vi "Serial_Init.vi"(8 "error in (no error)":errorcluster, 10 "input cluster":T1={"baud rate (9600)"=115200, "data bits (8)"=8, "parity (0:none)"=enum."None", "stop bits (10: 1 bit)"=10, "flow control (0:none)"=0, "termination char\n(0xA = '\\n' = LF) "=10, "Enable Termination\nChar (T)"=TRUE, "timeout (10sec)"=10000} {"termination char\n(0xA = '\\n' = LF)" format="%.0x"; "flow control (0:none)" items=["None", "XON/XOFF", "RTS/CTS", "XON/XOFF & RTS/CTS", "DTR/DSR", "XON/XOFF & DTR/DSR"]; "stop bits (10: 1 bit)" items=["1.0"=10, "1.5"=15, "2.0"=20]; "data bits (8)" min=5 max=8 step=1}, 11 "VISA Refnum in":refnum<visa-resource-name>="ASRL1::INSTR") -> (0 "error out":errorcluster, 1 "timeout (10sec)":u32=10000, 2 "Bytes at Port":u32, 3 "VISA Refnum out":refnum<visa-resource-name>)   [LabVIEW 2017]
uses:
  <vilib>/myRIO/Instrument Drivers/Onboard IO/UART/typedef/VISA Configuration.ctl
  <vilib>/Instr/_visa.llb/VISA Configure Serial Port (Instr).vi
  <vilib>/myRIO/Instrument Drivers/Onboard IO/UART/UART.lvlib
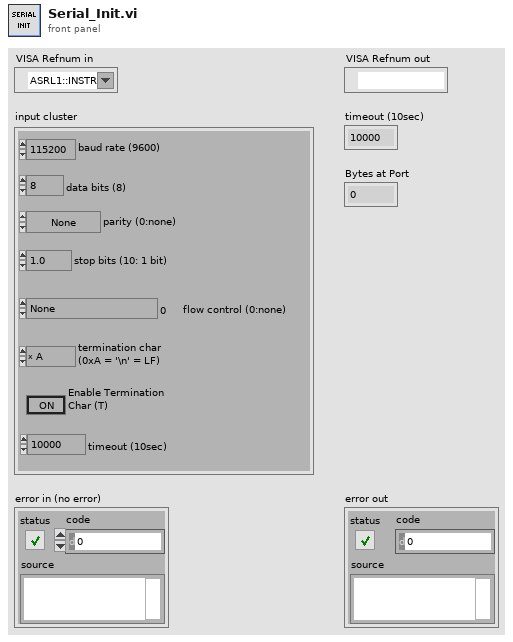
[diagram p1: front panel]
types:
  T1 = typedef "UART.lvlib/VISA Configuration.ctl" = cluster{"baud rate (9600)":u32, "data bits (8)":u16, "parity (0:none)":enum16{"None", "Odd", "Even", "Mark", "Space"}, "stop bits (10: 1 bit)":u16, "flow control (0:none)":u16, "termination char\n(0xA = '\\n' = LF) ":u8, "Enable Termination\nChar (T)":bool, "timeout (10sec)":u32}
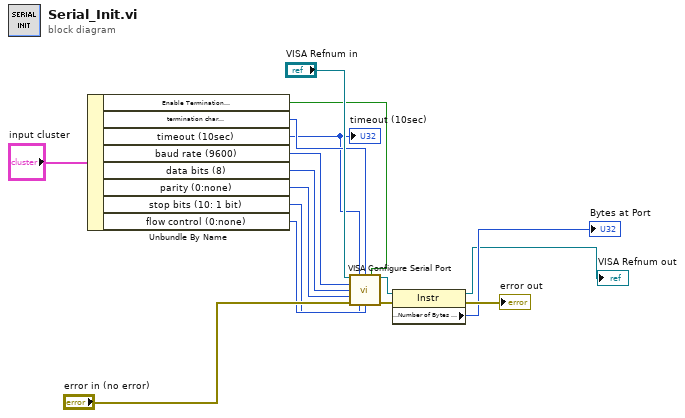
[diagram p0: block diagram]
diagram:
  n1 = Unbundle By Name("input cluster") -> ("Enable Termination\nChar (T)"=w8:bool, "termination char\n(0xA = '\\n' = LF)"=w7:u8, "timeout (10sec)"=w6:u32, "baud rate (9600)"=w1:u32, "data bits (8)"=w2:u16, "parity (0:none)"=w3:enum16{"None", "Odd", "Even", "Mark", "Space"}, "stop bits (10: 1 bit)"=w4:u16, "flow control (0:none)"=w5:u16)
  "timeout (10sec)" <- w6
  n2 = call-poly "VISA Configure Serial Port"("VISA resource name"="VISA Refnum in", "timeout (10sec)"=w6, "termination char\n(0xA = '\\n' = LF)"=w7, "Enable Termination\nChar (T)"=w8, "baud rate (9600)"=w1, "data bits (8)"=w2, "parity (0:none)"=w3, "error in (no error)"="error in (no error)", "stop bits (10: 1 bit)"=w4, "flow control (0:none)"=w5) -> ("VISA resource name out"=w12:refnum<visa-resource-name>, "error out"=w11:errorcluster)  [unwired: 4 in]
  n3 = property class="Instr"(reference=w12, error in=w11) -> (reference out=→"VISA Refnum out":refnum<visa-resource-name>, error out=→"error out":errorcluster, "Serial Settings:Number of Bytes at Serial Port"=→"Bytes at Port":u32)
